vi "AIM 664 test Load Frame Editor File.vi"(11 "file path (use dialog)":path) -> (0 "error out":errorcluster, 3 "data":T1[](array[typedef]) {"value"."Data" format="%.0x"; "value"."HeaderInfo"."NetSelect" items=["FDX_TX_FRAME_DLY_A"=0, "FDX_TX_FRAME_DLY_B"=1, "FDX_TX_FRAME_BOTH "=3, "FDX_TX_FRAME_ONLY_A"=4, "FDX_TX_FRAME_ONLY_B "=5]; "value"."HeaderInfo"."FrameStartMode" items=["FDX_TX_FRAME_START_IFG", "FDX_TX_FRAME_START_PGWT", "FDX_TX_FRAME_START_TRG"]; "value"."HeaderInfo"."PhysErrorInjection" items=["FDX_TX_FRAME_ERR_OFF"=0, "FDX_TX_FRAME_ERR_CRC"=1, "FDX_TX_FRAME_ERR_ALI"=2, "FDX_TX_FRAME_ERR_PRE"=4, "FDX_TX_FRAME_ERR_PHY"=8]; "value"."HeaderInfo"."SequenceNumberInit" items=["FDX_TX_FRAME_SEQ_INIT_AUTO"=65535]; "value"."HeaderInfo"."SequenceNumberOffset" items=["FDX_TX_FRAME_SEQ_OFFS_AUTO "=65535]; "value"."HeaderInfo"."PayloadGenerationMode" items=["FDX_TX_FRAME_PGM_USER"=0, "FDX_TX_FRAME_PGM_IP_PART"=1, "FDX_TX_FRAME_PGM_IP_FULL"=2, "FDX_TX_FRAME_PGM_IP_PART_TT"=10, "FDX_TX_FRAME_PGM_IP_FULL_TT"=20]; "value"."HeaderInfo"."PayloadBufferMode" items=["FDX_TX_FRAME_PBM_STD", "FDX_TX_FRAME_PBM_MAC", "FDX_TX_FRAME_PBM_UDP"]})   [LabVIEW 2020]
uses:
  Frame Configuration/controls/frame_file_entry.ctl
  Frame Configuration/controls/frame_record_type.ctl
  <instrlib>/AIM GmbH/_AIM 664/_controls/queue_header_generic.ctl
  <instrlib>/AIM GmbH/_AIM 664/AIM664LV.lvlib
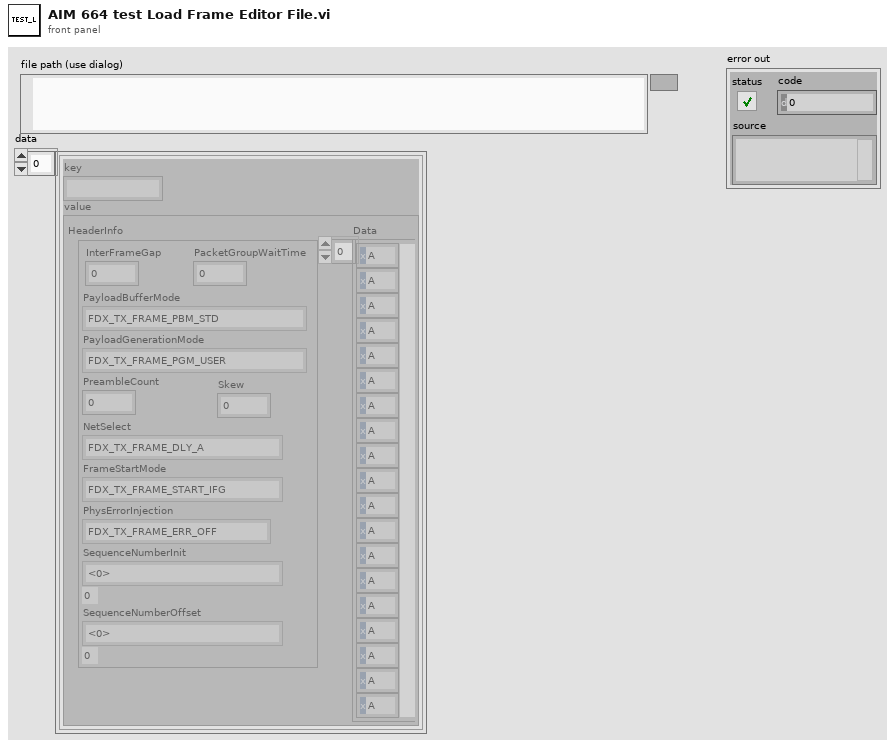
[diagram p1: front panel]
types:
  T1 = typedef "frame_file_entry.ctl" = cluster{"key":string, "value":T2}
  T2 = typedef "frame_record_type.ctl" = cluster{"HeaderInfo":T3, "Data":u8[]}
  T3 = typedef "AIM664LV.lvlib/queue_header_generic.ctl" = cluster{"InterFrameGap":u32, "PacketGroupWaitTime":u32, "PayloadBufferMode":u8, "PayloadGenerationMode":u8, "PreambleCount":u8, "Skew":u32, "NetSelect":u8, "FrameStartMode":u8, "PhysErrorInjection":u32, "SequenceNumberInit":u16, "SequenceNumberOffset":u16}
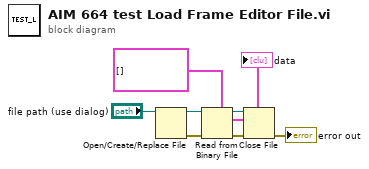
[diagram p0: block diagram]
diagram:
  n1 = Open/Create/Replace File(file path (use dialog)="file path (use dialog)") -> (refnum out=w5:refnum<file>, error out=w4:errorcluster)  [unwired: 5 in, 1 out]
  n2 = Read from Binary File(5:T1[] [] ("cluster"), 8:w4, 11:w5) -> (0:w6:errorcluster, 2:→"data":T1[], 3:w7:refnum<file>)  [unwired: 3 in, 1 out]
  n3 = Close File(refnum=w7, error in=w6) -> (error out=→"error out":errorcluster)  [unwired: 1 out]
